vi "Unload YAML Configuration.vi"(8 "Error In":errorcluster, 11 "YAML Handle In":u64) -> (0 "Error Out":errorcluster)   [LabVIEW 2019, in "YAML Config Reader.lvlib"]
uses:
  YAML Config Reader.lvlib
  target/debug/rust_labview_yaml.dll
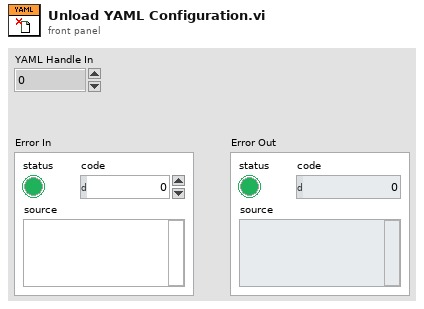
[diagram p1: front panel]
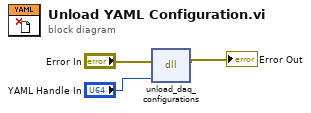
[diagram p0: block diagram]
diagram:
  n1 = dll-call lib="C:/dev/rust_labview_yaml/target/debug/rust_labview_yaml.dll" fn="unload_daq_configurations"(error in="Error In", "DaqConfigurations"="YAML Handle In") -> (error out=→"Error Out":errorcluster)  [unwired: 4 in, 1 out]
